vi "Process FCT Response.vi"(11 "FHPP in":refnum<class "FHPP.lvclass">) -> (3 "FHPP out":refnum<class "FHPP.lvclass">)   [LabVIEW 2022 SP3, in "FHPP.lvclass"]
uses:
  FHPP.lvclass
  FHPP.lvclass/FHPP.ctl
  TypeDefs/ResID.ctl
  TypeDefs/FCT Response.ctl
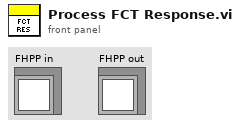
[diagram p1: front panel]
types:
  T1 = typedef "FHPP.lvclass/FCT Response.ctl" = cluster{"ResID":T2, "PNU":u16, "Subindex":u16, "Data":u32}
  T2 = typedef "FHPP.lvclass/ResID.ctl" = u8
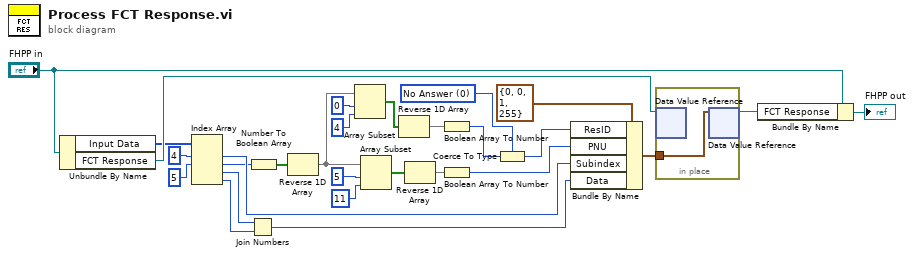
[diagram p0: block diagram]
diagram:
  w6 = T2 0 items=["No Answer"=0, "Parameter Transfered"=5, "Error"=7] ("ResID")
  n1 = Unbundle By Name("FHPP in") -> ("Input Data"=w15:u16[], "FCT Response"=w24:refnum<data-value>)
  n2 = Index Array(array=w15, index #1=4 ("index"), index #2=5 ("index")) -> (element #1=w20:u16, element #2=w14:u16, element #3=w21:u16, element #4=w22:u16)  [unwired: 2 in]
  n3 = Join Numbers(hi=w21, lo=w22) -> ((hi.lo)=w23:u32)
  n4 = Number To Boolean Array(number=w14) -> (Boolean array=w2:bool[])
  n5 = Reverse 1D Array(array=w2) -> (reversed array=w7:bool[])
  n6 = Array Subset(array=w7, index=0, length=4) -> (w4:bool[])
  n7 = Array Subset(array=w7, index=5, length=11) -> (w10:bool[])
  n8 = Reverse 1D Array(array=w4) -> (reversed array=w11:bool[])
  n9 = Reverse 1D Array(array=w10) -> (reversed array=w1:bool[])
  n10 = Boolean Array To Number(Boolean array=w11) -> (number=w5:u16)
  n11 = Boolean Array To Number(Boolean array=w1) -> (number=w18:u16)
  n12 = Coerce To Type(0:w5, 1:w6) -> (2:w17:T2)
  n13 = Bundle By Name(cluster=T1 {"ResID"=0, "PNU"=0, "Subindex"=1, "Data"=255} ("FCT Response"), "ResID"=w17, "PNU"=w18, "Subindex"=w20, "Data"=w23) -> (w25:T1)
  n14 = in-place {
    in-place-border: w25 -> [w29]
    n15 = in-place-dvr #1(w24) -> ()  [unwired: 2 out]
    n16 = in-place-dvr #1(w29) -> (w28:refnum<data-value>)  [unwired: 1 out]
  }
  n17 = Bundle By Name(cluster="FHPP in", "FCT Response"=w28) -> (→"FHPP out":refnum<class "FHPP.lvclass">)
